vi "Automatic-Approach-Retraction-MCL-2013-04-28-1a-data-storage-1b.vi"() -> ()   [LabVIEW 2012]
uses:
  <vilib>/rvi/eio/common/nirviEmuTemplateMethod_errors.vi
  <vilib>/rvi/Emulation/niFpgaSctlEmulationGetInTimedLoop.vi
  <vilib>/rvi/Emulation/niFpgaSctlEmulationGlobalWrite.vi
  <vilib>/rvi/interface/RandomDataEmulation/nirviRandomDataFPGAFIFO.vi
  <vilib>/rvi/interface/RandomDataEmulation/niFpgaRandomDataHandleErrors.vi
  <vilib>/eio/EIONode/EIONode.xnode
  <vilib>/rvi/DataTransferAndStorage/Container/XNode/niFpgaContainer.xnode
  <vilib>/rvi/interface/RandomDataEmulation/nirviRandomDataFpgaReadWriteTemplate.vi
  <vilib>/rvi/Analysis/measure/butterworth/XNode/niFpgaButterworthFilter.xnode
panel:
  out "TF-drift":i16
  out "Command Out":i16=-4104
  out "offset out":i16
  in  "provisional limit":i8=102
  in  "Steps per Feedback Region":i32=665
  out "accumulator limit":i8=-1
  in  "shift-divisions (always >=2)":i8=100
  out "limit indicator":u8
  in  "counter":i8 min=-1 step=1
  in  "I scale":i8=-1
  in  "PID gains (x 2^8)":T1={"proportional gain (Kc)"=1, "integral gain (Kc*Ts/Ti)"=0, "derivative gain (Kc*Td/Ts)"=0}
  in  "Internal Setpoint":i16=357
  in  "shift integrator":i32
  in  "P scale":i8=-1
  in  "Count(uSec)":u8=232
  in  "Stop Feedback Control":bool
  out "Tick Count(Ticks)":u32=3198398528
  in  "Data Acquisition Rate (usec)":u32=500000
  out "Data storage":bool=TRUE
  in  "Safetip Control ON/Off":bool
  out "Start Approach indicator":bool
  in  "safetip time wait":u32 caption="Count(uSec)"
  in  "Safetip retraction":u16
  out "safetip minimum indicator":bool
  out "Data counter":u16
  out "Counter Output":i16
  in  "Initial Position":i16
  in  "phase 1 control":bool
  in  "Manual Control":bool
  in  "Zposition MCL fine 2":i16
  in  "MCL counter 2":u16
  out "Curve indicator":u16
  in  "Number of curves":u16
  out "TF Freq shift":i16
  out "USBS Amplitude":i16
  in  "Timeout FIFO":i32=-1
  in  "Safetip Minimum":i16
  out "Phase 2":bool
  in  "Parameter":i16
  out "Phase 1":bool
  in  "Start Approach":bool
  out "MCL counter in range?":bool
  in  "Wait-tip-before-new-approach (usec)":u32
  in  "Fast Retraction After Cycle":i32
  in  "Wait-tip-before-approach":u32
  in  "Fast Retraction before approach":i32
  in  "Offset for Fast Approach":i16
  in  "Fast Approach (usec)":u32
  out "USBS Phase Signal":i16
  in  "Minimum for Approach Value":i16
  out "digital steps per region":u16
  in  "MCL Divisions":u16
  in  "MCL counter":u16
  in  "Fine Retraction (usec)":u32
  in  "TF at infinity":i16
  out "TF Phase Signal":i16(graph)
  out "Control Signal":i16
  out "MCL Sensor":i16
  in  "Fine Approach (usec)":u32
  in  "Setpoint Fine":i16
  out "Zposition MCL fine":i16
  in  "Initial Height (Fine)":i16=9113
types:
  T1 = cluster{"proportional gain (Kc)":i16, "integral gain (Kc*Ts/Ti)":i16, "derivative gain (Kc*Td/Ts)":i16}
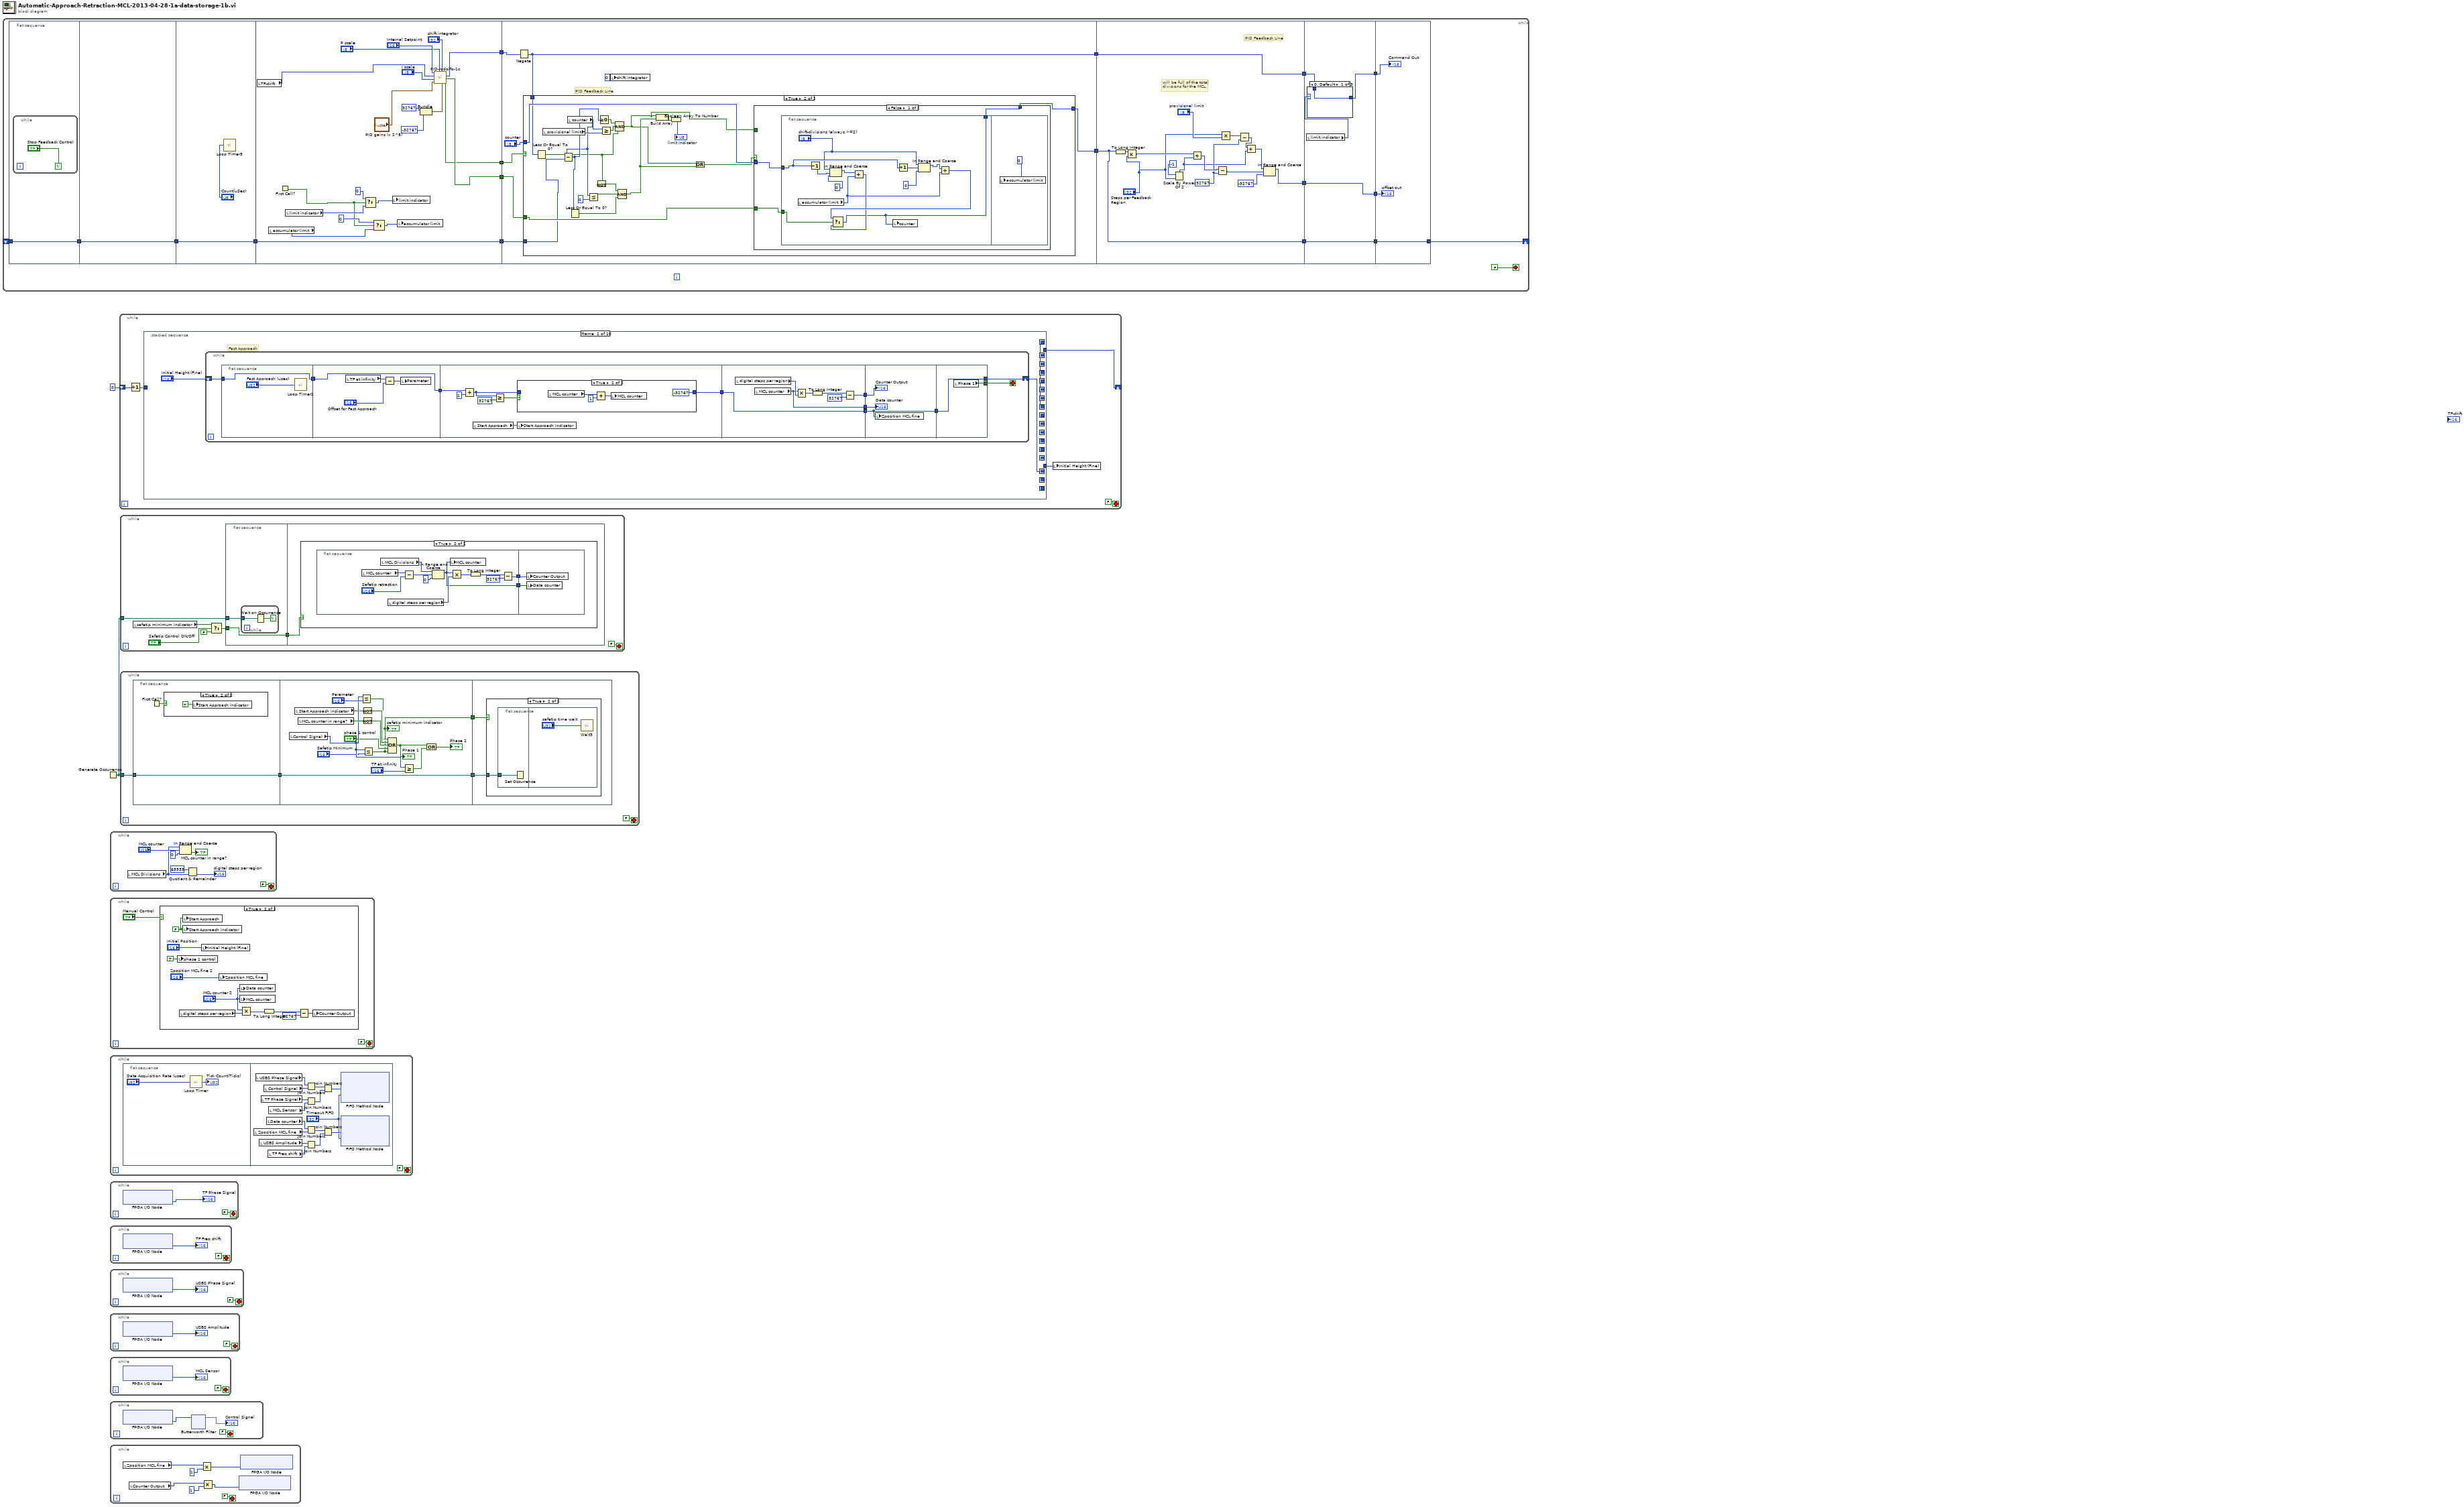
[diagram p0: block diagram]
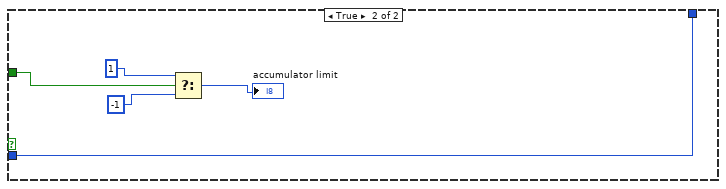
[diagram p3: hidden frame]
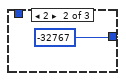
[diagram p4: hidden frame]
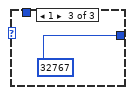
[diagram p5: hidden frame]
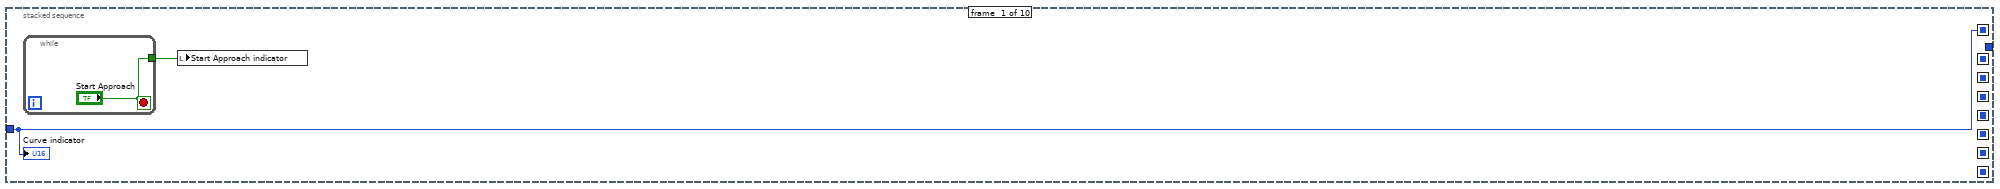
[diagram p10: hidden frame]
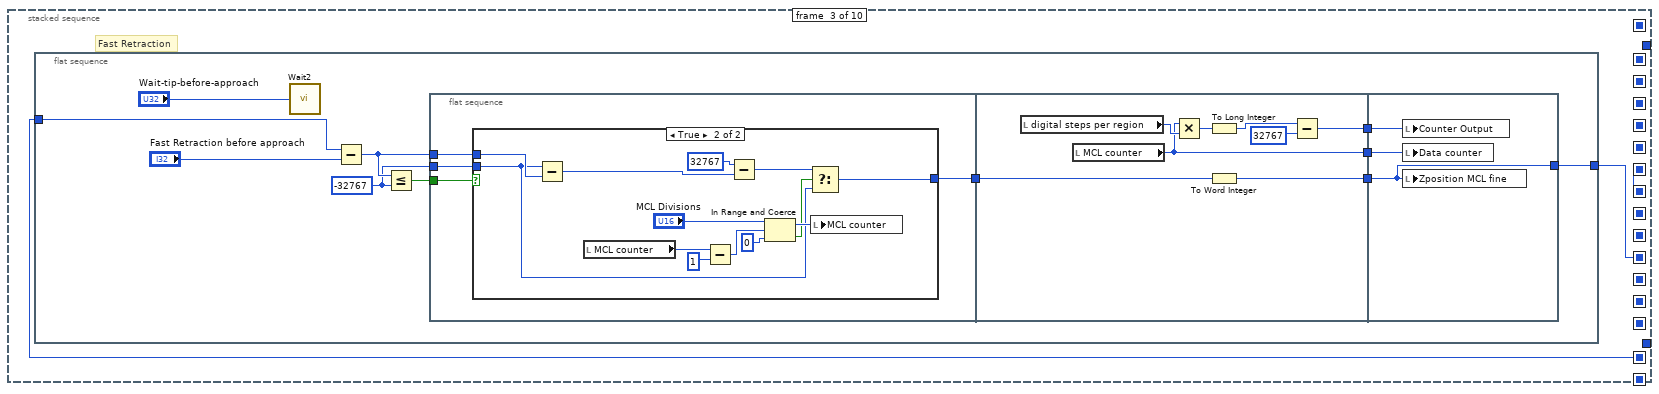
[diagram p12: hidden frame]
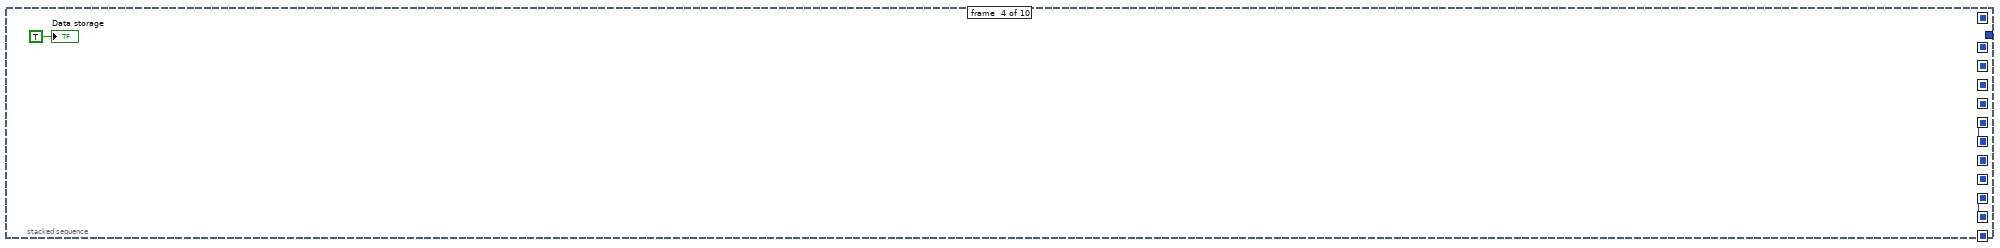
[diagram p14: hidden frame]
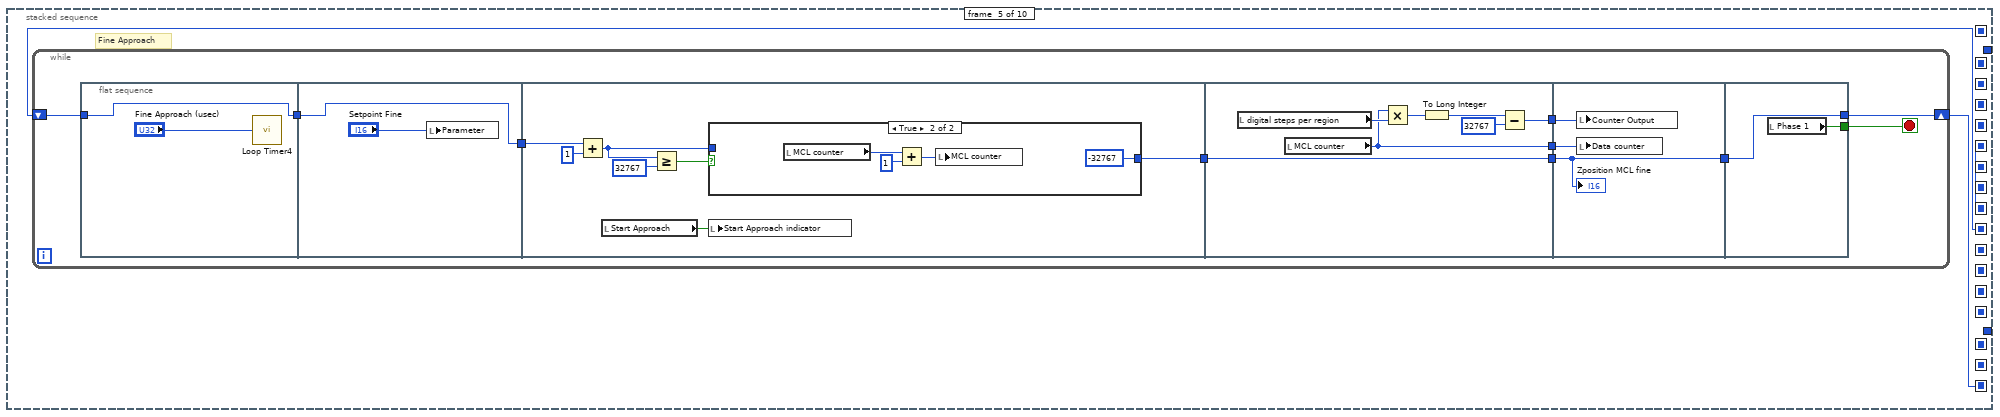
[diagram p15: hidden frame]
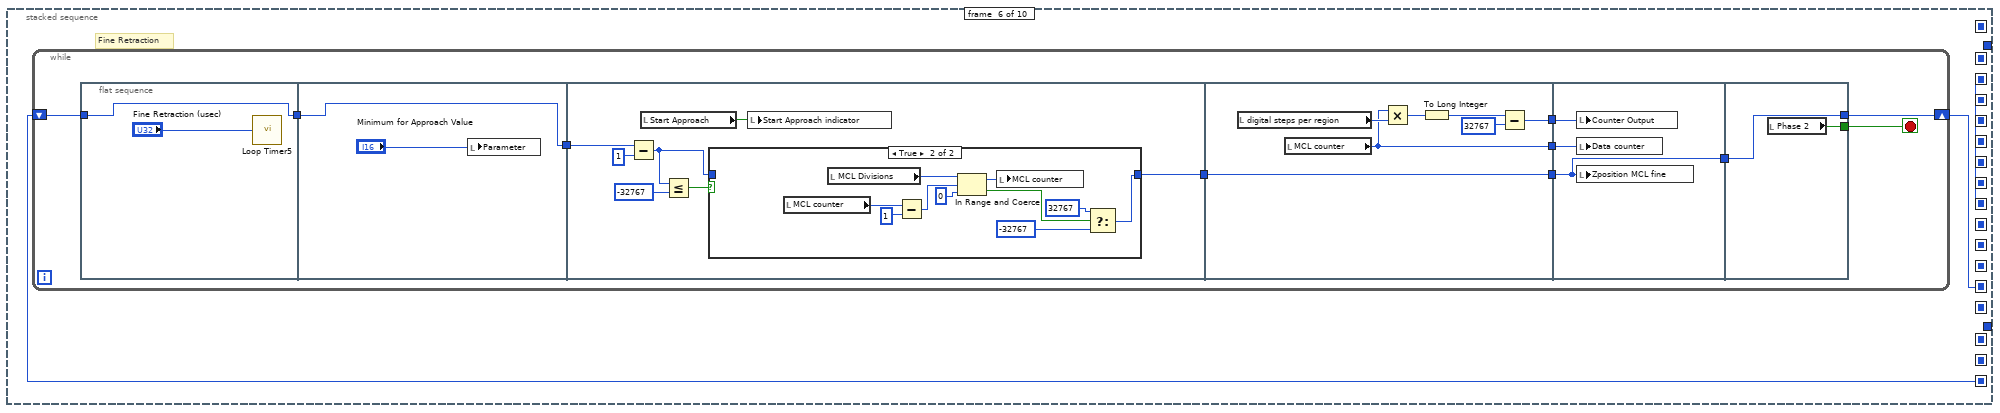
[diagram p17: hidden frame]
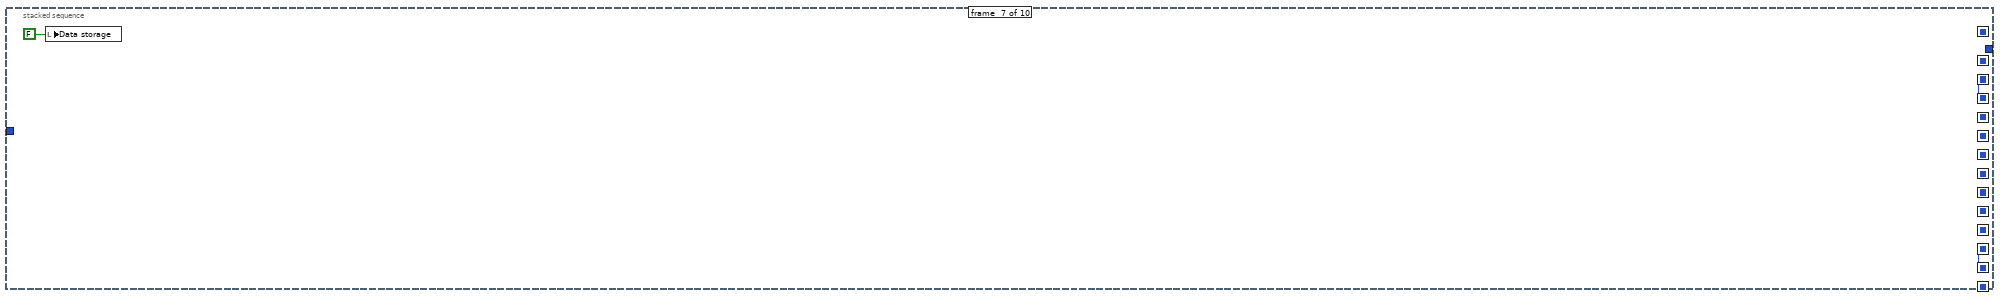
[diagram p19: hidden frame]
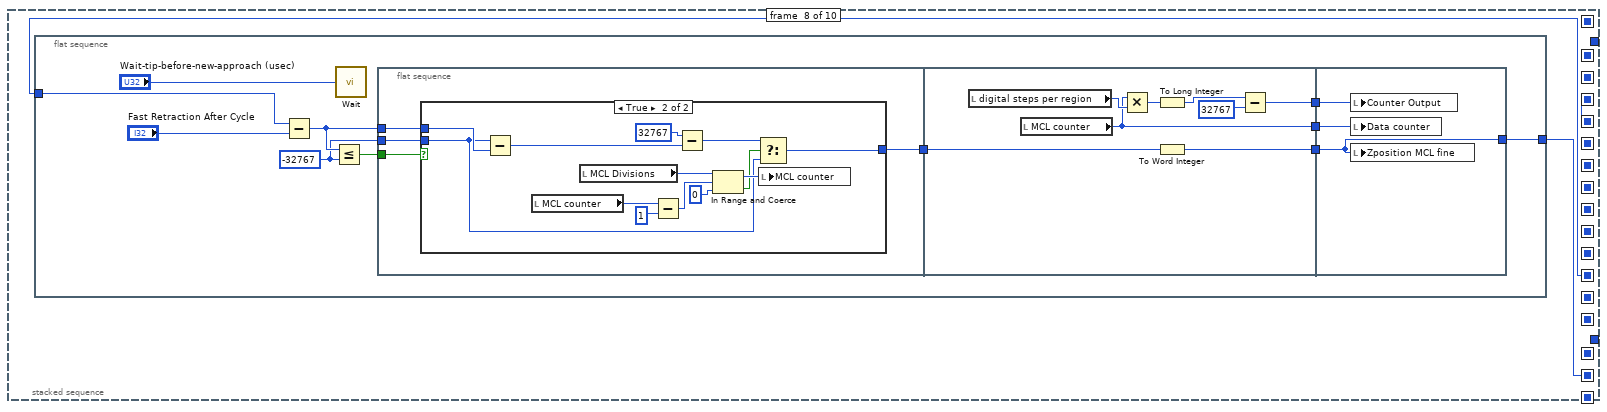
[diagram p20: hidden frame]
diagram:
  n1 = while {
    shift-right: [w11] -> _
    shift-left: _ -> [w10]
    stop <- FALSE stop-if-true
    n2 = flat-sequence {
      tunnel: w10 -> [w21]
      tunnel: [w21] -> w4
      tunnel: w4 -> [w23]
      tunnel: [w23] -> w3
      tunnel: [w24] -> w9
      tunnel: w3 -> [w24]
      tunnel: [w42] -> w8
      tunnel: [w41] -> w7
      tunnel: [w40] -> w6
      tunnel: w9 -> [w37]
      tunnel: [w37] -> w5
      tunnel: [w53] -> w14
      tunnel: w8 -> [w52]
      tunnel: [w48] -> w15
      tunnel: w7 -> [w50]
      tunnel: w6 -> [w49]
      tunnel: w5 -> [w47]
      tunnel: w15 -> [w110]
      tunnel: [w110] -> w17
      tunnel: w14 -> [w107]
      tunnel: [w108] -> w16
      tunnel: [w107] -> w13
      tunnel: [w114] -> w19
      tunnel: w17 -> [w116]
      tunnel: [w117] -> w18
      tunnel: w16 -> [w114]
      tunnel: w13 -> [w113]
      tunnel: [w113] -> w12
      tunnel: w19 -> [w121]
      tunnel: w18 -> [w123]
      tunnel: w12 -> [w122]
      tunnel: [w122] -> w11
      frame #0 {
        n3 = while {
          stop <- "Stop Feedback Control" continue-if-true
        }
      }
      frame #1 {
      }
      frame #2 {
        n4 = call "Loop Timer3"("Count(uSec)"="Count(uSec)") -> ()  [unwired: 1 out]
      }
      frame #3 {
        n5 = local read "TF-drift"() -> (w27:i16)
        n6 = local read "accumulator limit"() -> (w30:i8)
        n7 = First Call?() -> (First Call?: T/F=w28:bool)
        n8 = local read "limit indicator"() -> (w33:u8)
        n9 = Select(t=u8 0, s=w28, f=w33) -> (s? t:f=w34:u8)
        n10 = Select(t=i8 0, s=w28, f=w30) -> (s? t:f=w32:i8)
        n11 = local write "limit indicator"(w34) -> ()
        n12 = local write "accumulator limit"(w32) -> ()
        n13 = Bundle(i16 32767, i16 -32767) -> (w43:cluster{i16, i16})  [unwired: 1 in]
        n14 = call "PID-rodolfo-1c.vi"("output range"=w43, "shift integrator"="shift integrator", "P scale"="P scale", "PID gains (x 2^8)"="PID gains (x 2^8)", "I scale"="I scale", "process variable"=w27, "setpoint"="Internal Setpoint") -> ("yes/no"=w40:bool, "upper/lower"=w41:bool, "output"=w42:i16)  [unwired: 2 in]
      }
      frame #4 {
        # "PID Feedback Line"
        n15 = Negate(x=w52) -> (-x=w48:i16)
        n16 = case shown="True" w49 {
          tunnel: "counter" -> [w54 w74]
          tunnel: [w54 w73] -> w53
          tunnel: w50 -> [_ w57]
          tunnel: w48 -> [_ w62]
          tunnel: w47 -> [_ w55]
          frame False {
          }
          frame True {
            n17 = Less Or Equal To 0?(x=w62) -> (x <= 0?=w63:bool)
            n18 = local read "provisional limit"() -> (w70:i8)
            n19 = local read "counter"() -> (w65:i8)
            n20 = Subtract(x=w65, y=w55) -> (x-y=w66:i8)
            n21 = Less Or Equal To 0?(x=w66) -> (x <= 0?=w67:bool)
            n22 = Less Or Equal?(x=w65, y=u8 0) -> (x <= y?=w68:bool)
            n23 = Not(x=w63) -> (.not. x?=w64:bool)
            n24 = Greater Or Equal To 0?(x=w66) -> (x >= 0?=w72:bool)
            n25 = Greater Or Equal?(x=w65, y=w70) -> (x >= y?=w71:bool)
            n26 = Compound Arithmetic op=AND(w72, w71, w63) -> (w56:bool)
            n27 = Compound Arithmetic op=AND(w64, w68, w67) -> (w59:bool)
            n28 = Build Array(w56, w59) -> (w61:bool[])
            n29 = Boolean Array To Number(Boolean array=w61) -> (number=→"limit indicator":u8)
            n30 = Or(x=w56, y=w59) -> (x .or. y?=w58:bool)
            n31 = case shown="False" w58 {
              tunnel: w74 -> [w77 w96]
              tunnel: [w76 w96] -> w73
              tunnel: w57 -> [w75 _]
              tunnel: w56 -> [_ w92]
              frame False {
                n32 = flat-sequence {
                  tunnel: w77 -> [w83]
                  tunnel: [w80] -> w76
                  tunnel: w75 -> [w84]
                  frame #0 {
                    n33 = local read "accumulator limit"() -> (w79:i8)
                    n34 = Decrement(x=w83) -> (x-1=w87:i8)
                    n35 = In Range and Coerce(upper limit="shift-divisions (always >=2)", x=w87, lower limit=i8 0) -> (coerced(x)=w85:i8)  [unwired: 1 out]
                    n36 = Add(x=w85, y=w79) -> (x+y=w81:i8)
                    n37 = Increment(x=w83) -> (x+1=w88:i8)
                    n38 = In Range and Coerce(upper limit="shift-divisions (always >=2)", x=w88, lower limit=i8 0 ("y")) -> (coerced(x)=w90:i8)  [unwired: 1 out]
                    n39 = Add(x=w90, y=w79) -> (x+y=w82:i8)
                    n40 = Select(t=w82, s=w84, f=w81) -> (s? t:f=w80:i8)
                    n41 = local write "counter"(w80) -> ()
                  }
                  frame #1 {
                    n42 = local write "accumulator limit"(i8 0 ("accumulator limit")) -> ()
                  }
                }
              }
              frame True {
                n43 = Select(t=i8 1, s=w92, f=i8 -1) -> (s? t:f=→"accumulator limit":i8)
              }
            }
          }
        }
        n44 = local write "shift integrator"(0 ("new integrator")) -> ()
      }
      frame #5 {
        w100 = 32767 ("y")
        # "PID Feedback Line"
        # "will be full of the total\ndivisions for the MCL"
        n45 = To Long Integer(number=w107) -> (32bit integer=w106:i32)
        n46 = Multiply(x=w106, y="Steps per Feedback Region") -> (x*y=w111:i32)
        n47 = Scale By Power Of 2(n=i8 -1, x="Steps per Feedback Region") -> (x*2^n=w99:i32)
        n48 = Add(x=w111, y=w99) -> (x+y=w103:i32)
        n49 = Subtract(x=w103, y=w100) -> (x-y=w102:i32)
        n50 = Multiply(x="Steps per Feedback Region", y="provisional limit") -> (x*y=w101:i32)
        n51 = Subtract(x=w101, y=w100) -> (x-y=w98:i32)
        n52 = Add(x=w98, y=w99) -> (x+y=w97:i32)
        n53 = In Range and Coerce(upper limit=w97, x=w102, lower limit=-32767) -> (coerced(x)=w108:i32)  [unwired: 1 out]
      }
      frame #6 {
        n54 = local read "limit indicator"() -> (w115:u8)
        n55 = case shown="0, Default" w115 {
          tunnel: w116 -> [w118 _ _]
          tunnel: [w118 i16 -32767 i16 32767] -> w117
          frame 0, Default {
          }
          frame 2 {
          }
          frame 1 {
          }
        }
      }
      frame #7 {
        "Command Out" <- w123
        "offset out" <- w121
      }
    }
  }
  n56 = Generate Occurrence() -> (w1:refnum<k4>)
  n57 = while {
    stop <- FALSE stop-if-true
    n58 = local read "MCL Divisions"() -> (w124:u16)
    n59 = In Range and Coerce(upper limit=w124, x="MCL counter", lower limit=u16 0) -> (In Range?=→"MCL counter in range?":bool)  [unwired: 1 out]
    n60 = Quotient & Remainder(x=65535, y=w124) -> (floor(x/y)=→"digital steps per region":i32)  [unwired: 1 out]
  }
  n61 = while {
    stop <- FALSE stop-if-true
    n62 = case shown="True" "Manual Control" {
      frame False {
      }
      frame True {
        w133 = FALSE ("Start Approach")
        n63 = local write "phase 1 control"(TRUE ("phase 1 control")) -> ()
        n64 = local read "digital steps per region"() -> (w139:u16)
        n65 = local write "Start Approach"(w133) -> ()
        n66 = local write "Start Approach indicator"(w133) -> ()
        n67 = local write "Initial Height (Fine)"("Initial Position") -> ()
        n68 = local write "Zposition MCL fine"("Zposition MCL fine 2") -> ()
        n69 = local write "Data counter"("MCL counter 2") -> ()
        n70 = local write "MCL counter"("MCL counter 2") -> ()
        n71 = Multiply(x="MCL counter 2", y=w139) -> (x*y=w135:u16)
        n72 = To Long Integer(number=w135) -> (32bit integer=w134:i32)
        n73 = Subtract(x=w134, y=32767) -> (x-y=w137:i32)
        n74 = local write "Counter Output"(w137) -> ()
      }
    }
  }
  n75 = while {
    stop <- FALSE stop-if-true
    n76 = flat-sequence {
      frame #0 {
        n77 = call "Loop Timer"("Count(Ticks)"="Data Acquisition Rate (usec)") -> ("Tick Count(Ticks)"=→"Tick Count(Ticks)":u32)
      }
      frame #1 {
        n78 = local read "Zposition MCL fine"() -> (w156:i16)
        n79 = local read "USBS Phase Signal"() -> (w151:i16)
        n80 = local read "USBS Amplitude"() -> (w147:i16)
        n81 = local read "TF Phase Signal"() -> (w149:i16)
        n82 = local read "Control Signal"() -> (w150:i16)
        n83 = local read "Data counter"() -> (w157:u16)
        n84 = local read "TF Freq shift"() -> (w146:i16)
        n85 = local read "MCL Sensor"() -> (w148:i16)
        n86 = Join Numbers(hi=w151, lo=w150) -> ((hi.lo)=w159:u32)
        n87 = Join Numbers(hi=w149, lo=w148) -> ((hi.lo)=w160:u32)
        n88 = Join Numbers(hi=w157, lo=w156) -> ((hi.lo)=w154:u32)
        n89 = Join Numbers(hi=w147, lo=w146) -> ((hi.lo)=w155:u32)
        n90 = Join Numbers(hi=w159, lo=w160) -> ((hi.lo)=w158:u64)
        n91 = Join Numbers(hi=w154, lo=w155) -> ((hi.lo)=w153:u64)
        n92 = xnode ("FIFO Method Node")("Element"=w158, "Timeout"="Timeout FIFO") -> ()  [unwired: 1 in, 2 out]
        n93 = xnode ("FIFO Method Node")("Element"=w153, "Timeout"="Timeout FIFO") -> ()  [unwired: 1 in, 2 out]
      }
    }
  }
  n94 = while {
    stop <- FALSE stop-if-true
    n95 = xnode "FPGA I/O Node"() -> ("Connector0/AI1"=→"TF Phase Signal":i16)  [unwired: 1 in, 1 out]
  }
  n96 = while {
    stop <- FALSE stop-if-true
    n97 = xnode "FPGA I/O Node"() -> ("Connector0/AI2"=→"TF Freq shift":i16)  [unwired: 1 in, 1 out]
  }
  n98 = while {
    stop <- FALSE stop-if-true
    n99 = xnode "FPGA I/O Node"() -> ("Connector0/AI4"=→"USBS Phase Signal":i16)  [unwired: 1 in, 1 out]
  }
  n100 = while {
    stop <- FALSE stop-if-true
    n101 = xnode "FPGA I/O Node"() -> ("Connector0/AI5"=→"USBS Amplitude":i16)  [unwired: 1 in, 1 out]
  }
  n102 = while {
    stop <- FALSE stop-if-true
    n103 = xnode "FPGA I/O Node"() -> ("Connector0/AI6"=→"MCL Sensor":i16)  [unwired: 1 in, 1 out]
  }
  n104 = while {
    stop <- FALSE stop-if-true
    n105 = xnode "FPGA I/O Node"() -> ("Connector0/AI7"=w172:i16)  [unwired: 1 in, 1 out]
    n106 = xnode "Butterworth Filter"("input data"=w172) -> ("output data"=→"Control Signal":fxp<+/-,20,20>)  [unwired: 2 in]
  }
  n107 = while {
    stop <- FALSE stop-if-true
    n108 = local read "Zposition MCL fine"() -> (w186:i16)
    n109 = local read "Counter Output"() -> (w182:i16)
    n110 = Multiply(x=w186, y=i16 1) -> (x*y=w185:i16)
    n111 = Multiply(x=w182, y=i16 1) -> (x*y=w183:i16)
    n112 = xnode "FPGA I/O Node"("Connector0/AO2"=w183) -> ()  [unwired: 1 in, 1 out]
    n113 = xnode "FPGA I/O Node"("Connector0/AO7"=w185) -> ()  [unwired: 1 in, 1 out]
  }
  n114 = while {
    shift-right: [w189] -> _
    shift-left: u16 0 ("t") -> [w188]
    stop <- FALSE stop-if-true
    n115 = Increment(x=w188) -> (x+1=w190:u16)
    n116 = stacked-sequence {
      seq-local: [w194 _ _ _ _ _ _ _ _ _] -> [_ w197 _ _ _ _ _ _ _ _]
      seq-local: [_ w198 _ _ _ _ _ _ _ _] -> [_ _ w241 _ _ _ _ _ _ _]
      seq-local: [_ w197 _ _ _ _ _ _ _ _] -> [_ _ w239 _ _ _ _ _ _ _]
      seq-local: [_ _ w240 _ _ _ _ _ _ _] -> [_ _ _ w284 _ _ _ _ _ _]
      seq-local: [_ _ w239 _ _ _ _ _ _ _] -> [_ _ _ w283 _ _ _ _ _ _]
      seq-local: [_ _ _ w284 _ _ _ _ _ _] -> [_ _ _ _ w287 _ _ _ _ _]
      seq-local: [_ _ _ w283 _ _ _ _ _ _] -> [_ _ _ _ w285 _ _ _ _ _]
      seq-local: [_ _ _ _ w286 _ _ _ _ _] -> [_ _ _ _ _ w328 _ _ _ _]
      seq-local: [_ _ _ _ w285 _ _ _ _ _] -> [_ _ _ _ _ w326 _ _ _ _]
      seq-local: [_ _ _ _ _ w327 _ _ _ _] -> [_ _ _ _ _ _ w375 _ _ _]
      seq-local: [_ _ _ _ _ w326 _ _ _ _] -> [_ _ _ _ _ _ w374 _ _ _]
      seq-local: [_ _ _ _ _ _ w375 _ _ _] -> [_ _ _ _ _ _ _ w378 _ _]
      seq-local: [_ _ _ _ _ _ w374 _ _ _] -> [_ _ _ _ _ _ _ w376 _ _]
      seq-local: [_ _ _ _ _ _ _ w377 _ _] -> [_ _ _ _ _ _ _ _ w424 _]
      seq-local: [_ _ _ _ _ _ _ w376 _ _] -> [_ _ _ _ _ _ _ _ w419 _]
      seq-local: [_ _ _ _ _ _ _ _ w424 _] -> [_ _ _ _ _ _ _ _ _ w427]
      seq-local: [_ _ _ _ _ _ _ _ w420 _] -> [_ _ _ _ _ _ _ _ _ w426]
      tunnel: w190 -> [w194 _ _ _ _ _ _ _ _ _]
      tunnel: [_ _ _ _ _ _ _ _ _ w427] -> w192
      tunnel: [_ _ _ _ _ _ _ _ _ w426] -> w189
      frame #0 {
        n117 = while {
          tunnel: ["Start Approach"] -> w193
          stop <- "Start Approach" stop-if-true
        }
        n118 = local write "Start Approach indicator"(w193) -> ()
        "Curve indicator" <- w194
      }
      frame #1 {
        # "Fast Approach"
        n119 = while {
          shift-right: [w207] -> w198
          shift-left: "Initial Height (Fine)" -> [w208]
          stop <- w203 stop-if-true
          n120 = flat-sequence {
            tunnel: w208 -> [w210]
            tunnel: [w210] -> w205
            tunnel: [w214] -> w206
            tunnel: w205 -> [w214]
            tunnel: [w220] -> w202
            tunnel: w206 -> [w221]
            tunnel: w202 -> [w233]
            tunnel: [w233] -> w201
            tunnel: [w230] -> w200
            tunnel: [w229] -> w199
            tunnel: w201 -> [w236]
            tunnel: [w236] -> w204
            tunnel: w200 -> [w235]
            tunnel: w199 -> [w234]
            tunnel: [w238] -> w207
            tunnel: w204 -> [w238]
            tunnel: [w237] -> w203
            frame #0 {
              n121 = call "Loop Timer2"("Count(uSec)"="Fast Approach (usec)") -> ()  [unwired: 1 out]
            }
            frame #1 {
              n122 = local read "TF at infinity"() -> (w211:i16)
              n123 = Subtract(x=w211, y="Offset for Fast Approach") -> (x-y=w213:i16)
              n124 = local write "Parameter"(w213) -> ()
            }
            frame #2 {
              n125 = Add(x=w221, y=i16 1) -> (x+y=w216:i16)
              n126 = local read "Start Approach"() -> (w215:bool)
              n127 = Greater Or Equal?(x=w216, y=i16 32767) -> (x >= y?=w217:bool)
              n128 = case shown="True" w217 {
                tunnel: [w222 i16 -32767] -> w220
                tunnel: w216 -> [w222 _]
                frame False {
                }
                frame True {
                  n129 = local read "MCL counter"() -> (w224:u16)
                  n130 = Add(x=w224, y=u16 1) -> (x+y=w223:u16)
                  n131 = local write "MCL counter"(w223) -> ()
                }
              }
              n132 = local write "Start Approach indicator"(w215) -> ()
            }
            frame #3 {
              n133 = local read "digital steps per region"() -> (w232:u16)
              n134 = local read "MCL counter"() -> (w229:u16)
              n135 = Multiply(x=w229, y=w232) -> (x*y=w228:u16)
              n136 = To Long Integer(number=w228) -> (32bit integer=w227:i32)
              n137 = Subtract(x=w227, y=32767) -> (x-y=w230:i32)
            }
            frame #4 {
              n138 = local write "Zposition MCL fine"(w236) -> ()
              "Counter Output" <- w235
              "Data counter" <- w234
            }
            frame #5 {
              n139 = local read "Phase 1"() -> (w237:bool)
            }
          }
        }
      }
      frame #2 {
        # "Fast Retraction"
        n140 = flat-sequence {
          tunnel: [w248] -> w240
          tunnel: w241 -> [w249]
          frame #0 {
            w246 = -32767 ("y")
            n141 = call "Wait2"("Count(uSec)"="Wait-tip-before-approach") -> ()  [unwired: 1 out]
            n142 = Subtract(x=w249, y="Fast Retraction before approach") -> (x-y=w251:i32)
            n143 = Less Or Equal?(x=w251, y=w246) -> (x <= y?=w252:bool)
            n144 = flat-sequence {
              tunnel: w252 -> [w256]
              tunnel: w251 -> [w255]
              tunnel: w246 -> [w253]
              tunnel: [w254] -> w245
              tunnel: w245 -> [w274]
              tunnel: [w273] -> w244
              tunnel: [w275] -> w243
              tunnel: [w276] -> w242
              tunnel: [w281] -> w248
              tunnel: w244 -> [w281]
              tunnel: w243 -> [w280]
              tunnel: w242 -> [w279]
              frame #0 {
                n145 = case shown="True" w256 {
                  tunnel: w255 -> [w257 w267]
                  tunnel: [w257 w259] -> w254
                  tunnel: w253 -> [_ w258]
                  frame False {
                  }
                  frame True {
                    n146 = Subtract(x=w258, y=w267) -> (x-y=w266:i32)
                    n147 = local read "MCL counter"() -> (w270:u16)
                    n148 = Subtract(x=w270, y=u16 1) -> (x-y=w263:u16)
                    n149 = Subtract(x=32767, y=w266) -> (x-y=w260:i32)
                    n150 = In Range and Coerce(upper limit="MCL Divisions", x=w263, lower limit=u16 0 ("upper limit")) -> (coerced(x)=w262:u16, In Range?=w261:bool)
                    n151 = Select(t=w260, s=w261, f=w258) -> (s? t:f=w259:i32)
                    n152 = local write "MCL counter"(w262) -> ()
                  }
                }
              }
              frame #1 {
                n153 = local read "digital steps per region"() -> (w278:u16)
                n154 = local read "MCL counter"() -> (w275:u16)
                n155 = Multiply(x=w275, y=w278) -> (x*y=w272:u16)
                n156 = To Long Integer(number=w272) -> (32bit integer=w271:i32)
                n157 = To Word Integer(number=w274) -> (16bit integer=w273:i16)
                n158 = Subtract(x=w271, y=32767) -> (x-y=w276:i32)
              }
              frame #2 {
                n159 = local write "Counter Output"(w279) -> ()
                n160 = local write "Data counter"(w280) -> ()
                n161 = local write "Zposition MCL fine"(w281) -> ()
              }
            }
          }
        }
      }
      frame #3 {
        "Data storage" <- TRUE
      }
      frame #4 {
        # "Fine Approach"
        n162 = while {
          shift-right: [w296] -> w286
          shift-left: w287 -> [w297]
          stop <- w288 stop-if-true
          n163 = flat-sequence {
            tunnel: w297 -> [w299]
            tunnel: [w299] -> w294
            tunnel: [w301] -> w295
            tunnel: w294 -> [w301]
            tunnel: [w307] -> w293
            tunnel: w295 -> [w308]
            tunnel: w293 -> [w320]
            tunnel: [w320] -> w292
            tunnel: [w317] -> w291
            tunnel: [w316] -> w290
            tunnel: w292 -> [w321]
            tunnel: w291 -> [w323]
            tunnel: w290 -> [w322]
            tunnel: [w321] -> w289
            tunnel: [w325] -> w296
            tunnel: w289 -> [w325]
            tunnel: [w324] -> w288
            frame #0 {
              n164 = call "Loop Timer4"("Count(uSec)"="Fine Approach (usec)") -> ()  [unwired: 1 out]
            }
            frame #1 {
              n165 = local write "Parameter"("Setpoint Fine") -> ()
            }
            frame #2 {
              n166 = Add(x=w308, y=i16 1) -> (x+y=w303:i16)
              n167 = local read "Start Approach"() -> (w302:bool)
              n168 = Greater Or Equal?(x=w303, y=i16 32767) -> (x >= y?=w304:bool)
              n169 = case shown="True" w304 {
                tunnel: [w309 i16 -32767] -> w307
                tunnel: w303 -> [w309 _]
                frame False {
                }
                frame True {
                  n170 = local read "MCL counter"() -> (w310:u16)
                  n171 = Add(x=w310, y=u16 1) -> (x+y=w312:u16)
                  n172 = local write "MCL counter"(w312) -> ()
                }
              }
              n173 = local write "Start Approach indicator"(w302) -> ()
            }
            frame #3 {
              n174 = local read "digital steps per region"() -> (w319:u16)
              n175 = local read "MCL counter"() -> (w316:u16)
              n176 = Multiply(x=w316, y=w319) -> (x*y=w315:u16)
              n177 = To Long Integer(number=w315) -> (32bit integer=w314:i32)
              n178 = Subtract(x=w314, y=32767) -> (x-y=w317:i32)
            }
            frame #4 {
              n179 = local write "Counter Output"(w323) -> ()
              n180 = local write "Data counter"(w322) -> ()
              "Zposition MCL fine" <- w321
            }
            frame #5 {
              n181 = local read "Phase 1"() -> (w324:bool)
            }
          }
        }
      }
      frame #5 {
        # "Fine Retraction"
        n182 = while {
          shift-right: [w337] -> w327
          shift-left: w328 -> [w338]
          stop <- w331 stop-if-true
          n183 = flat-sequence {
            tunnel: w338 -> [w340]
            tunnel: [w340] -> w334
            tunnel: [w342] -> w335
            tunnel: w334 -> [w342]
            tunnel: [w348] -> w336
            tunnel: w335 -> [w349]
            tunnel: w336 -> [w367]
            tunnel: [w367] -> w333
            tunnel: [w362] -> w330
            tunnel: [w361] -> w329
            tunnel: w333 -> [w368]
            tunnel: [w368] -> w332
            tunnel: w330 -> [w370]
            tunnel: w329 -> [w369]
            tunnel: [w372] -> w337
            tunnel: w332 -> [w372]
            tunnel: [w371] -> w331
            frame #0 {
              n184 = call "Loop Timer5"("Count(uSec)"="Fine Retraction (usec)") -> ()  [unwired: 1 out]
            }
            frame #1 {
              n185 = local write "Parameter"("Minimum for Approach Value") -> ()
            }
            frame #2 {
              n186 = Subtract(x=w349, y=i16 1) -> (x-y=w344:i16)
              n187 = local read "Start Approach"() -> (w343:bool)
              n188 = Less Or Equal?(x=w344, y=i16 -32767) -> (x <= y?=w346:bool)
              n189 = case shown="True" w346 {
                tunnel: w344 -> [w350 _]
                tunnel: [w350 w351] -> w348
                frame False {
                }
                frame True {
                  n190 = local read "MCL counter"() -> (w360:u16)
                  n191 = local read "MCL Divisions"() -> (w358:u16)
                  n192 = Subtract(x=w360, y=u16 1) -> (x-y=w356:u16)
                  n193 = In Range and Coerce(upper limit=w358, x=w356, lower limit=u16 0) -> (coerced(x)=w355:u16, In Range?=w354:bool)
                  n194 = local write "MCL counter"(w355) -> ()
                  n195 = Select(t=i16 32767, s=w354, f=i16 -32767) -> (s? t:f=w351:i16)
                }
              }
              n196 = local write "Start Approach indicator"(w343) -> ()
            }
            frame #3 {
              n197 = local read "digital steps per region"() -> (w366:u16)
              n198 = local read "MCL counter"() -> (w362:u16)
              n199 = Multiply(x=w362, y=w366) -> (x*y=w364:u16)
              n200 = To Long Integer(number=w364) -> (32bit integer=w363:i32)
              n201 = Subtract(x=w363, y=32767) -> (x-y=w361:i32)
            }
            frame #4 {
              n202 = local write "Counter Output"(w369) -> ()
              n203 = local write "Data counter"(w370) -> ()
              n204 = local write "Zposition MCL fine"(w368) -> ()
            }
            frame #5 {
              n205 = local read "Phase 2"() -> (w371:bool)
            }
          }
        }
      }
      frame #6 {
        n206 = local write "Data storage"(FALSE ("Data storage")) -> ()
      }
      frame #7 {
        n207 = flat-sequence {
          tunnel: [w385] -> w377
          tunnel: w378 -> [w386]
          frame #0 {
            w383 = -32767 ("y")
            n208 = Subtract(x=w386, y="Fast Retraction After Cycle") -> (x-y=w389:i32)
            n209 = Less Or Equal?(x=w389, y=w383) -> (x <= y?=w388:bool)
            n210 = call "Wait"("Count(uSec)"="Wait-tip-before-new-approach (usec)") -> ()  [unwired: 1 out]
            n211 = flat-sequence {
              tunnel: w389 -> [w393]
              tunnel: w388 -> [w392]
              tunnel: w383 -> [w390]
              tunnel: [w391] -> w382
              tunnel: w382 -> [w411]
              tunnel: [w410] -> w381
              tunnel: [w413] -> w380
              tunnel: [w412] -> w379
              tunnel: [w417] -> w385
              tunnel: w381 -> [w417]
              tunnel: w380 -> [w418]
              tunnel: w379 -> [w416]
              frame #0 {
                n212 = case shown="True" w392 {
                  tunnel: w393 -> [w394 w405]
                  tunnel: [w394 w395] -> w391
                  tunnel: w390 -> [_ w396]
                  frame False {
                  }
                  frame True {
                    n213 = Subtract(x=w396, y=w405) -> (x-y=w404:i32)
                    n214 = local read "MCL counter"() -> (w407:u16)
                    n215 = local read "MCL Divisions"() -> (w401:u16)
                    n216 = Subtract(x=w407, y=u16 1) -> (x-y=w402:u16)
                    n217 = Subtract(x=32767, y=w404) -> (x-y=w397:i32)
                    n218 = In Range and Coerce(upper limit=w401, x=w402, lower limit=u16 0) -> (coerced(x)=w399:u16, In Range?=w398:bool)
                    n219 = Select(t=w397, s=w398, f=w396) -> (s? t:f=w395:i32)
                    n220 = local write "MCL counter"(w399) -> ()
                  }
                }
              }
              frame #1 {
                n221 = local read "digital steps per region"() -> (w415:u16)
                n222 = local read "MCL counter"() -> (w412:u16)
                n223 = Multiply(x=w412, y=w415) -> (x*y=w409:u16)
                n224 = To Long Integer(number=w409) -> (32bit integer=w408:i32)
                n225 = To Word Integer(number=w411) -> (16bit integer=w410:i16)
                n226 = Subtract(x=w408, y=32767) -> (x-y=w413:i32)
              }
              frame #2 {
                n227 = local write "Counter Output"(w418) -> ()
                n228 = local write "Data counter"(w416) -> ()
                n229 = local write "Zposition MCL fine"(w417) -> ()
              }
            }
          }
        }
      }
      frame #8 {
        n230 = Less?(x=w419, y="Number of curves") -> (x < y?=w422:bool)
        n231 = local write "Start Approach"(w422) -> ()
        n232 = Select(t=w419, s=w422, f=u16 0 ("t")) -> (s? t:f=w420:u16)
      }
      frame #9 {
        "Start Approach indicator" <- TRUE ("Start Approach indicator")
      }
    }
    n233 = local write "Initial Height (Fine)"(w192) -> ()
  }
  n234 = while {
    tunnel: w1 -> [w430]
    stop <- FALSE stop-if-true
    n235 = local read "safetip minimum indicator"() -> (w433:bool)
    n236 = Select(t=w433, s="Safetip Control ON/Off", f=FALSE) -> (s? t:f=w428:bool)
    n237 = flat-sequence {
      tunnel: w430 -> [w436]
      tunnel: [w435] -> w429
      tunnel: w428 -> [w435]
      tunnel: w429 -> [w439]
      frame #0 {
        n238 = while {
          tunnel: w436 -> [w437]
          stop <- w438 continue-if-true
          n239 = Wait on Occurrence(2:w437) -> (0:w438:bool)  [unwired: 2 in]
        }
      }
      frame #1 {
        n240 = case shown="True" w439 {
          frame False {
          }
          frame True {
            n241 = flat-sequence {
              tunnel: [w446] -> w441
              tunnel: [w442] -> w440
              tunnel: w441 -> [w454]
              tunnel: w440 -> [w453]
              frame #0 {
                n242 = local read "MCL counter"() -> (w450:u16)
                n243 = local read "MCL Divisions"() -> (w449:u16)
                n244 = local read "digital steps per region"() -> (w452:u16)
                n245 = Subtract(x=w450, y="Safetip retraction") -> (x-y=w447:u16)
                n246 = In Range and Coerce(upper limit=w449, x=w447, lower limit=u16 0) -> (coerced(x)=w446:u16)  [unwired: 1 out]
                n247 = local write "MCL counter"(w446) -> ()
                n248 = Multiply(x=w446, y=w452) -> (x*y=w445:u16)
                n249 = To Long Integer(number=w445) -> (32bit integer=w444:i32)
                n250 = Subtract(x=w444, y=32767) -> (x-y=w442:i32)
              }
              frame #1 {
                n251 = local write "Counter Output"(w453) -> ()
                n252 = local write "Data counter"(w454) -> ()
              }
            }
          }
        }
      }
    }
  }
  n253 = while {
    tunnel: w1 -> [w457]
    stop <- FALSE stop-if-true
    n254 = flat-sequence {
      tunnel: [w460] -> w458
      tunnel: w457 -> [w460]
      tunnel: [w465] -> w456
      tunnel: w458 -> [w463]
      tunnel: [w463] -> w455
      tunnel: w456 -> [w479]
      tunnel: w455 -> [w478]
      frame #0 {
        n255 = First Call?() -> (First Call?: T/F=w461:bool)
        n256 = case shown="True" w461 {
          frame False {
          }
          frame True {
            n257 = local write "Start Approach indicator"(TRUE ("Start Approach indicator")) -> ()
          }
        }
      }
      frame #1 {
        n258 = local read "Control Signal"() -> (w469:i16)
        n259 = local read "Start Approach indicator"() -> (w464:bool)
        n260 = local read "MCL counter in range?"() -> (w476:bool)
        n261 = Less Or Equal?(x=w469, y="Parameter") -> (x <= y?=w474:bool)
        n262 = Not(x=w464) -> (.not. x?=w475:bool)
        n263 = Not(x=w476) -> (.not. x?=w477:bool)
        n264 = Less Or Equal?(x=w469, y="Safetip Minimum") -> (x <= y?=w465:bool)
        "safetip minimum indicator" <- w465
        n265 = Compound Arithmetic op=OR(w474, w475, w477, "phase 1 control", w465) -> (w466:bool)
        "Phase 1" <- w466
        n266 = Greater Or Equal?(x=w469, y="TF at infinity") -> (x >= y?=w471:bool)
        n267 = Compound Arithmetic op=OR(w466, w471) -> (→"Phase 2":bool)
      }
      frame #2 {
        n268 = case shown="True" w479 {
          tunnel: w478 -> [_ w480]
          frame False {
          }
          frame True {
            n269 = flat-sequence {
              tunnel: w480 -> [w481]
              frame #0 {
                n270 = Set Occurrence(w481) -> ()
              }
              frame #1 {
                n271 = call "Wait3"("Count(uSec)"="safetip time wait") -> ()  [unwired: 1 out]
              }
            }
          }
        }
      }
    }
  }
